vi "IMU Serial Read.vi"(8 "Invert Polarity?":bool, 9 "data bits (8)":i32=8 min=5 max=8 step=1, 10 "stop bits (10: 1 bit)":u16(ring)=10 items=["1.0"=10, "1.5"=15, "2.0"=20], 11 "baud rate (230400)":u32=230400) -> ()   [LabVIEW 2016]
uses:
  <vilib>/rvi/Emulation/niFpgaGetClockAttributes.vi
  <vilib>/rvi/Emulation/niFpgaSctlEmulationGetInTimedLoop.vi
  <vilib>/rvi/Emulation/niFpgaEmulationReportErrorSimple.vi
  <vilib>/rvi/eio/common/nirviEmuTemplateMethod_errors.vi
  <vilib>/rvi/Emulation/niFpgaCriticalErrorInLSC.vi
  <vilib>/rvi/Emulation/niFpgaProcessEmulError.vi
  <vilib>/rvi/Emulation/niFpgaEmulationIsFPGAContextNoSignature.vi
  <vilib>/rvi/errors/niFpgaSetErrorForExecOnDevCompSimple.vi
  <vilib>/rvi/eio/common/nirviEmuReportErrorAndStop.vi
  <vilib>/rvi/DataTransferAndStorage/Container/Common/niFpgaContainerGetUniqueNameForEmu.vi
  <vilib>/rvi/FIFO/Fifo_Resource/nirvififoEmulationSetSize.vi
  <vilib>/rvi/FIFO/Fifo_Resource/nirviFifoEmulationQueueMgr.vi
  <instcachedir>/0/nirviFifoEmulationQueueMgr_E5CAEC123FF24DC58D834DCA3CDAA9B5.lvgen/nirviFifoEmulationQueueMgr_E5CAEC123FF24DC58D834DCA3CDAA9B5_000.vi
  <vilib>/rvi/FIFO/Fifo_Resource/nirvififoEmulationDetermineInputValidOut.vi
  <vilib>/rvi/FIFO/Fifo_Resource/nirvififoEmulationCreateLock.vi
  <vilib>/rvi/FIFO/Fifo_Resource/nirvififoEmulationObtainLock.vi
  <vilib>/rvi/FIFO/Fifo_Resource/nirvififoEmulationReleaseLock.vi
  <vilib>/rvi/occurrence/nirviWaitOnOccurrenceBase.vi
  <vilib>/rvi/errors/nirviReportUnexpectedCaseInternalError.vi
  <vilib>/rvi/errors/nirviReportUnexpectedCaseInternalError (U32).vi
  <vilib>/eio/EIONode/EIONode.xnode
  <vilib>/rvi/DataTransferAndStorage/Container/XNode/niFpgaContainer.xnode
  <vilib>/rvi/FIFO/Fifo_Resource/nirvififoEmulationWrite.vi
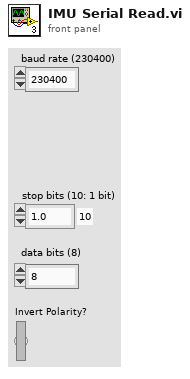
[diagram p1: front panel]
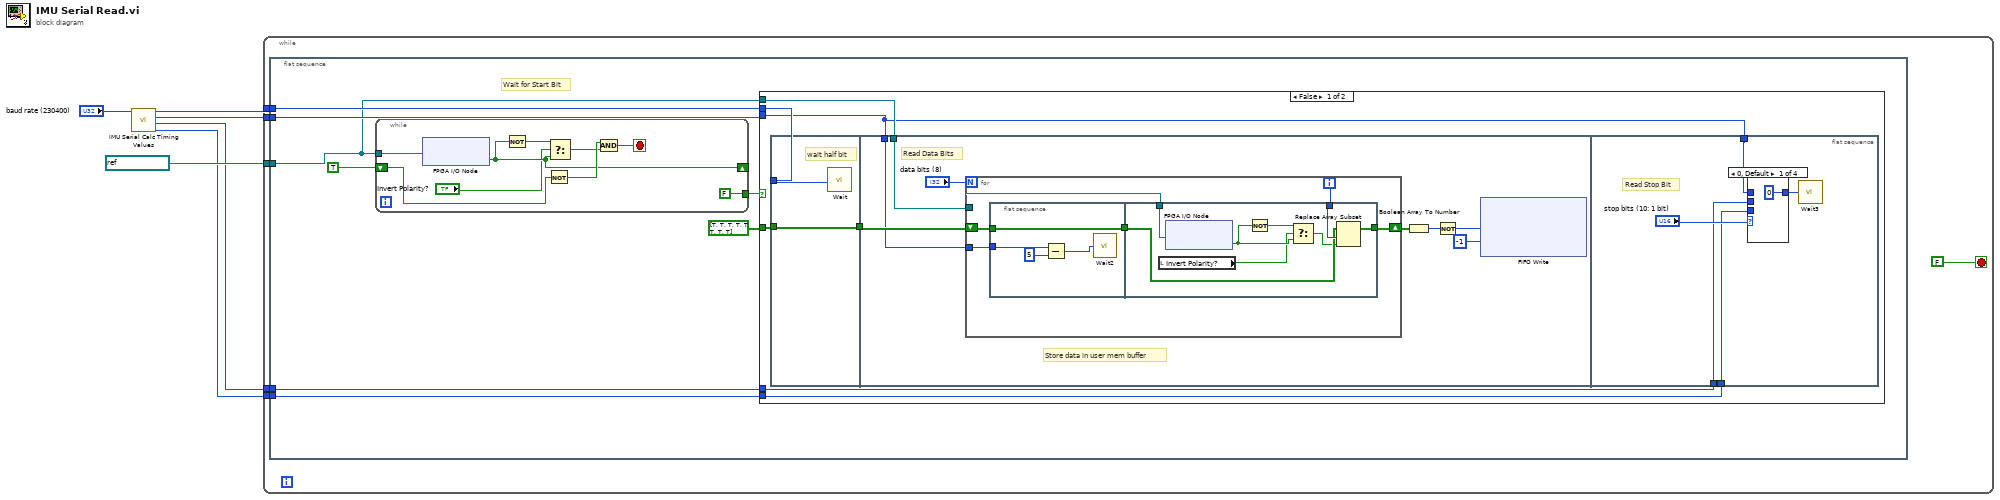
[diagram p0: block diagram]
diagram:
  n1 = call "IMU Serial Calc Timing Values.vi"("baud rate (1000000)"="baud rate (230400)") -> ("Two Bit"=w2:u32, "One and Half Bit"=w3:u32, "One Bit"=w4:u32, "Half Bit"=w5:u32)  [unwired: 3 in]
  n2 = while {
    tunnel: w2 -> [w12]
    tunnel: w3 -> [w11]
    tunnel: w4 -> [w10]
    tunnel: w5 -> [w9]
    tunnel: refnum<k21> "MXP/DIO9" ("Receive") -> [w8]
    stop <- FALSE stop-if-true
    n3 = flat-sequence {
      tunnel: w12 -> [w19]
      tunnel: w11 -> [w18]
      tunnel: w10 -> [w17]
      tunnel: w9 -> [w16]
      tunnel: w8 -> [w13]
      frame #0 {
        # "Wait for Start Bit"
        n4 = while {
          tunnel: [FALSE] -> w15
          shift-right: [w67] -> _
          shift-left: TRUE -> [w72]
          tunnel: w13 -> [w70]
          stop <- w65 stop-if-true
          n5 = xnode "FPGA I/O Node"("FPGA I/O In"=w70) -> ("I/O Item"=w67:bool)  [unwired: 1 out]
          n6 = Not(x=w67) -> (.not. x?=w69:bool)
          n7 = Not(x=w72) -> (.not. x?=w71:bool)
          n8 = Select(t=w69, s="Invert Polarity?", f=w67) -> (s? t:f=w68:bool)
          n9 = And(x=w71, y=w68) -> (x .and. y?=w65:bool)
        }
        n10 = case shown="False" w15 {
          tunnel: bool[] [TRUE, TRUE, TRUE, TRUE, TRUE, TRUE, TRUE, TRUE] -> [w27 _]
          tunnel: w16 -> [w26 _]
          tunnel: w17 -> [w24 _]
          tunnel: w18 -> [w22 _]
          tunnel: w19 -> [w23 _]
          tunnel: w13 -> [w25 _]
          frame False {
            n11 = flat-sequence {
              tunnel: [w29] -> w21
              tunnel: w27 -> [w29]
              tunnel: w26 -> [w28]
              tunnel: w24 -> [w36]
              tunnel: w25 -> [w32]
              tunnel: w21 -> [w37]
              tunnel: w22 -> [w57]
              tunnel: w23 -> [w58]
              tunnel: w24 -> [w59]
              frame #0 {
                # "wait half bit"
                n12 = call "Wait"("Count(Ticks)"=w28) -> ()  [unwired: 1 out]
              }
              frame #1 {
                # "Store data in user mem buffer"
                # "Read Data Bits"
                n13 = for {
                  N: "data bits (8)" -> [_]
                  shift-right: [w40] -> w35
                  shift-left: w37 -> [w43]
                  tunnel: w36 -> [w41]
                  tunnel: w32 -> [w38]
                  i -> [w39]
                  n14 = flat-sequence {
                    tunnel: w43 -> [w47]
                    tunnel: [w47] -> w42
                    tunnel: w41 -> [w46]
                    tunnel: w39 -> [w55]
                    tunnel: w42 -> [w54]
                    tunnel: [w53] -> w40
                    tunnel: w38 -> [w52]
                    frame #0 {
                      n15 = Subtract(x=w46, y=u32 5 ("SecondTune")) -> (x-y=w45:u32)
                      n16 = call "Wait2"("Count(Ticks)"=w45) -> ()  [unwired: 1 out]
                    }
                    frame #1 {
                      n17 = local read "Invert Polarity?"() -> (w48:bool)
                      n18 = xnode "FPGA I/O Node"("FPGA I/O In"=w52) -> ("I/O Item"=w49:bool)  [unwired: 1 out]
                      n19 = Not(x=w49) -> (.not. x?=w51:bool)
                      n20 = Select(t=w51, s=w48, f=w49) -> (s? t:f=w50:bool)
                      n21 = Replace Array Subset(array=w54, new element=w50, index=w55) -> (w53:bool[])
                    }
                  }
                }
                n22 = Boolean Array To Number(Boolean array=w35) -> (number=w34:u8)
                n23 = Not(x=w34) -> (.not. x?=w31:u8)
                n24 = xnode ("FIFO Write")("Element"=w31, "Timeout"=-1) -> ()  [unwired: 1 in, 2 out]
              }
              frame #2 {
                # "Read Stop Bit"
                n25 = case shown="0, Default" "stop bits (10: 1 bit)" {
                  tunnel: w59 -> [_ w62 _ _]
                  tunnel: w57 -> [_ _ w63 _]
                  tunnel: w58 -> [_ _ _ w64]
                  tunnel: [u32 0 ("One Bit") w62 w63 w64] -> w56
                  frame 0, Default {
                  }
                  frame 10 {
                  }
                  frame 15 {
                  }
                  frame 20 {
                  }
                }
                n26 = call "Wait3"("Count(Ticks)"=w56) -> ()  [unwired: 1 out]
              }
            }
          }
          frame True {
          }
        }
      }
    }
  }
